vi "niLvFpgaNotchCU(16-bit)(n-chan).vi"(0 "filter state in":i32[](array[numeric])=[0, 0, 0], 1 "reset":bool, 5 "input data":i16, 7 "accumulator in":i32, 9 "adder in":i32, 11 "iteration":u8) -> (4 "filter state out":i32, 6 "state to multiply":i32, 8 "accumulator out":i32, 10 "adder out":i32, 15 "terminate":bool)   [LabVIEW 2017]
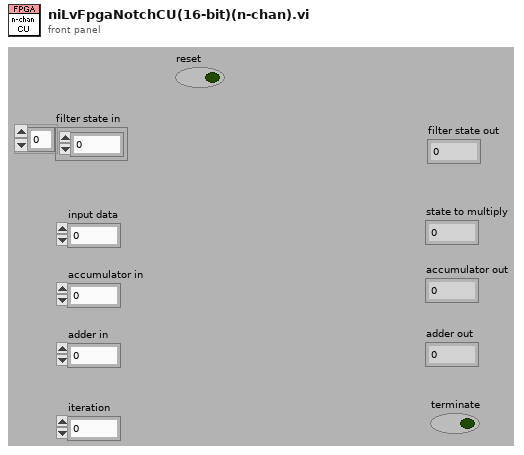
[diagram p1: front panel]
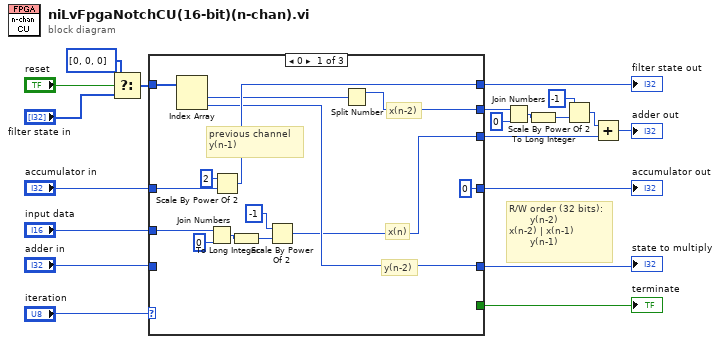
[diagram p0: block diagram]
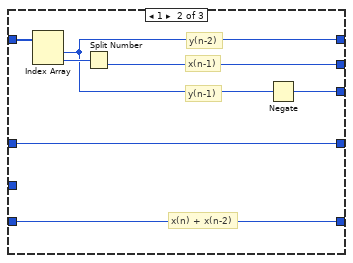
[diagram p2: hidden frame]
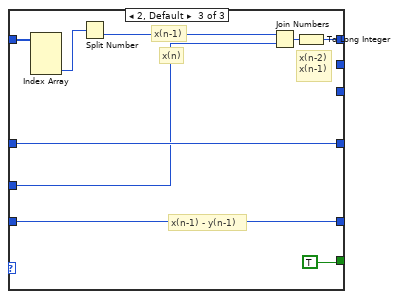
[diagram p3: hidden frame]
diagram:
  # "R/W order (32 bits):\n       y(n-2)\nx(n-2) | x(n-1)\n       y(n-1)"
  n1 = Select(t=i32[] [0, 0, 0], s="reset", f="filter state in") -> (s? t:f=w8:i32[])
  n2 = case shown="0" "iteration" {
    tunnel: "input data" -> [w23 _ w42]
    tunnel: [w22 w38 _] -> w20
    tunnel: "adder in" -> [_ w39 w49]
    tunnel: [w28 w39 w49] -> w13
    tunnel: "accumulator in" -> [w33 w41 w50]
    tunnel: [0 ("Numeric") w41 w50] -> w12
    tunnel: [_ _ TRUE] -> w18
    tunnel: [w30 w35 w44] -> w14
    tunnel: w8 -> [w31 w40 w43]
    tunnel: [w27 w36 _] -> w4
    frame 0 {
      # "previous channel \ny(n-1)"
      # "x(n)"
      # "x(n-2)"
      # "y(n-2)"
      n3 = Index Array(array=w31) -> (element #1=w29:i32, element #2=w28:i32)  [unwired: 2 in]
      n4 = Join Numbers(hi=w23, lo=i16 0) -> ((hi.lo)=w24:u32)
      n5 = Scale By Power Of 2(n=2, x=w33) -> (x*2^n=w30:i32)
      n6 = To Long Integer(number=w24) -> (32bit integer=w26:i32)
      n7 = Scale By Power Of 2(n=-1, x=w26) -> (x*2^n=w22:i32)
      n8 = Split Number(x=w29) -> (hi(x)=w27:u16)  [unwired: 1 out]
    }
    frame 1 {
      # "y(n-1)"
      # "y(n-2)"
      # "x(n-1)"
      # "x(n) + x(n-2)"
      n9 = Index Array(array=w40) -> (element #1=w35:i32, element #2=w37:i32)  [unwired: 2 in]
      n10 = Split Number(x=w37) -> (lo(x)=w36:u16)  [unwired: 1 out]
      n11 = Negate(x=w35) -> (-x=w38:i32)
    }
    frame 2, Default {
      # "x(n)"
      # "x(n-1)"
      # "x(n-2)\nx(n-1)"
      # "x(n-1) - y(n-1)"
      n12 = Index Array(array=w43) -> (element #3=w46:i32)  [unwired: 3 in, 2 out]
      n13 = Split Number(x=w46) -> (lo(x)=w45:u16)  [unwired: 1 out]
      n14 = Join Numbers(hi=w45, lo=w42) -> ((hi.lo)=w47:u32)
      n15 = To Long Integer(number=w47) -> (32bit integer=w44:i32)
    }
  }
  "state to multiply" <- w13
  "terminate" <- w18
  "accumulator out" <- w12
  "filter state out" <- w14
  n16 = Join Numbers(hi=w4, lo=i16 0) -> ((hi.lo)=w6:u32)
  n17 = To Long Integer(number=w6) -> (32bit integer=w2:i32)
  n18 = Scale By Power Of 2(n=-1, x=w2) -> (x*2^n=w3:i32)
  n19 = Add(x=w3, y=w20) -> (x+y=→"adder out":i32)
